vi "AI_Oblicz mnozniki teoret.vi"(6 "Mnozniki":dbl[][](array[numeric]), 8 "error in (no error)":errorcluster, 10 "AI param aktywne in":T1[](array[typedef]) {"Numer" min=1 max=8 step=1}, 11 "Aktywne Array in":bool[](array[boolean])) -> (0 "error out":errorcluster, 1 "Mnożniki out":dbl[](array[numeric]), 2 "AI param aktywne out":T1[](array[typedef]) {"Numer" min=1 max=8 step=1}, 3 "Aktywne Array out":bool[](array[boolean]), 4 "Mnożniki wszystkie out":dbl[](array[numeric]))   [LabVIEW 2014]
doc: "Oblicza teoretyczny mnożnik\ndla każdego zakresu"
uses:
  Kontrolki/GUI/AI_parametry.ctl
  Kontrolki/GUI/AI_wartosc.ctl
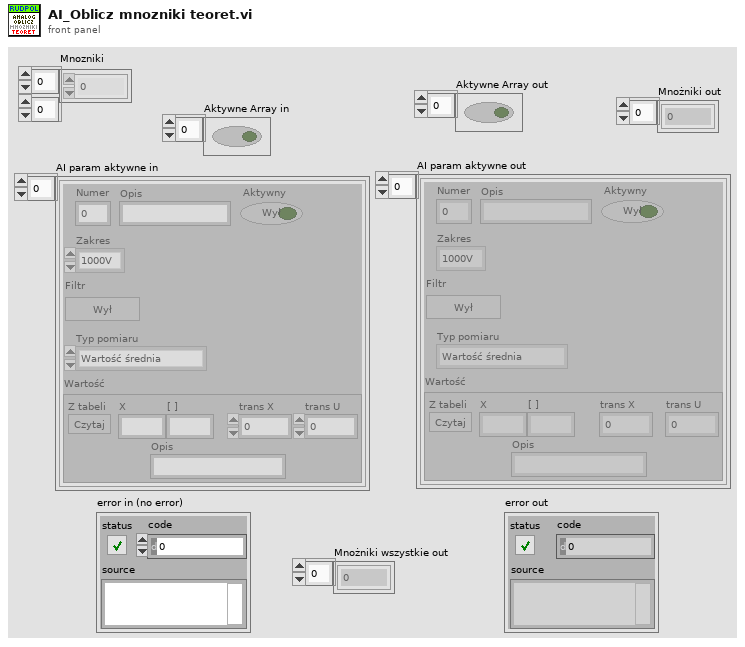
[diagram p1: front panel]
types:
  T1 = typedef "AI_parametry.ctl" = cluster{"Numer":u8, "Opis":string, "Zakres":enum16{"1000V", "300V", "30V", "3V", "0,3V"}, "Filtr":bool, "Typ pomiaru":enum16{"Wartość średnia", "Średnia wyprostowana", "Wartość skuteczna"}, "Aktywny":bool, "Wartość":T2}
  T2 = typedef "AI_wartosc.ctl" = cluster{"X":string, "[ ]":string, "trans X":dbl, "trans U":dbl, "Z tabeli":bool, "Opis":string}
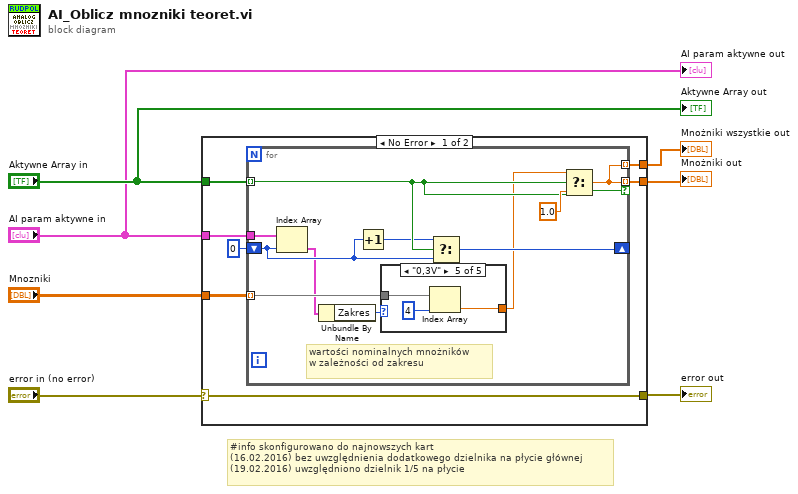
[diagram p0: block diagram]
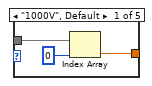
[diagram p2: hidden frame]
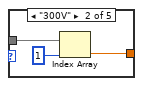
[diagram p3: hidden frame]
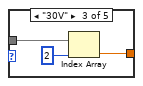
[diagram p4: hidden frame]
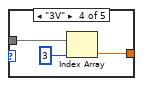
[diagram p5: hidden frame]
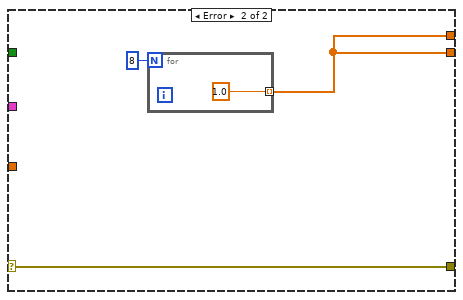
[diagram p6: hidden frame]
diagram:
  # "#info skonfigurowano do najnowszych kart\n(16.02.2016) bez uwzględnienia dodatkowego dzielnika na płycie głównej\n(19.02.2016) uwzględniono dzielnik 1/5 na płycie"
  n1 = case shown="No Error" "error in (no error)" {
    selector: "error in (no error)" -> [w11 w43]
    tunnel: "AI param aktywne in" -> [w13 _]
    tunnel: "Aktywne Array in" -> [w12 _]
    tunnel: [w11 w43] -> w5
    tunnel: [w10 w41] -> w4
    tunnel: [w9 w41] -> w3
    tunnel: "Mnozniki" -> [w8 _]
    frame No Error {
      n2 = for {
        tunnel: w12 -> [w23] mode=indexing
        tunnel: w13 -> [w24]
        shift-right: [w22] -> _
        shift-left: 0 -> [w20]
        tunnel: [w19] -> w10 mode=indexing if=w23
        tunnel: [w19] -> w9 mode=indexing
        tunnel: w8 -> [w17] mode=indexing
        # "wartości nominalnych mnożników\nw zależności od zakresu"
        n3 = Index Array(array=w24, index=w20) -> (element=w16:T1)
        n4 = Unbundle By Name(w16) -> ("Zakres"=w18:enum16{"1000V", "300V", "30V", "3V", "0,3V"})
        n5 = Increment(x=w20) -> (x+1=w21:i32)
        n6 = case shown="\"0,3V\"" w18 {
          tunnel: [w27 w29 w33 w35 w38] -> w15
          tunnel: w17 -> [w28 w30 w32 w36 w39]
          frame "1000V", Default {
            n7 = Index Array(array=w28, index=0) -> (element=w27:dbl)
          }
          frame "300V" {
            n8 = Index Array(array=w30, index=1) -> (element=w29:dbl)
          }
          frame "30V" {
            n9 = Index Array(array=w32, index=2) -> (element=w33:dbl)
          }
          frame "3V" {
            n10 = Index Array(array=w36, index=3) -> (element=w35:dbl)
          }
          frame "0,3V" {
            n11 = Index Array(array=w39, index=4) -> (element=w38:dbl)
          }
        }
        n12 = Select(t=w21, s=w23, f=w20) -> (s? t:f=w22:i32)
        n13 = Select(t=w15, s=w23, f=1.0) -> (s? t:f=w19:dbl)
      }
    }
    frame Error {
      n14 = for {
        N: 8 -> [_]
        tunnel: [1.0] -> w41 mode=indexing
      }
    }
  }
  "error out" <- w5
  "Mnożniki out" <- w4
  "Mnożniki wszystkie out" <- w3
  "Aktywne Array out" <- "Aktywne Array in"
  "AI param aktywne out" <- "AI param aktywne in"
